vi "Backup.vi"() -> ()   [LabVIEW 2020, in "Backup.lvlib"]
uses:
  Backup.lvlib
  Seiten/System Einstellungen V2/Aktioen FGV System Konstanten.ctl
  Sprachverwaltung/FGV Aktion Tabelle zerlegen.ctl
  Seiten/FT-IR/Span/Aktion FGV Span.ctl
  Bildwechsel/Bild-Auswahl.ctl
  <vilib>/Platform/browser.llb/Open URL in Default Browser (path).vi
  Allgemein/allgemeine Sub-VIs.lvlib
  Seiten/System Einstellungen V2/System Einstellungen V2.lvlib
  Bildwechsel/Bildwechsel.lvlib
  Seiten/FT-IR/Span/Spanfaktor.lvlib
  Sprachverwaltung/Sprachverwaltung.lvlib
panel:
  out "Statusanzeige":string
  out "SysLog":bool
  out "recipes":bool caption="Rezepte"
  out "Communication":bool caption="Kommunikation"
  out "cRIO KonfigIAG":bool
  out "cRIO startup":bool
  in  "Listenfeld":i32(listbox)
  in  "Cancel":bool
  in  "Backup":bool caption="Update"
  # "Backup Manager"
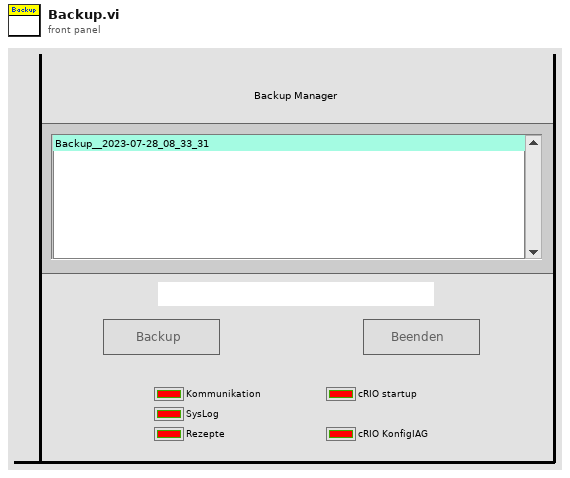
[diagram p1: front panel]
types:
  T1 = typedef "Sprachverwaltung.lvlib/FGV Aktion Tabelle zerlegen.ctl" = enum16{"laden", "vereinzeln", "speichern"}
  T2 = enum8{"Enabled", "Disabled", "Disabled and Grayed Out"}
  T3 = typedef "System Einstellungen V2.lvlib/Aktioen FGV System Konstanten.ctl" = enum16{"lesen", "laden", "speichern", "Sprache"}
  T4 = typedef "FT-IR.lvlib/Spanfaktor.lvlib/Aktion FGV Span.ctl" = enum16{"lesen", "Span", "Seite aktiv", "Offset", "FGV aktualisiert", "Aktualisierung aufheben"}
  T5 = typedef "Bildwechsel.lvlib/Bild-Auswahl.ctl" = enum16{"lesen", "Initialisieren", "Beenden", "Grafik", "Anlagenübersicht", "Anlagengrenzwerte", "Log Konfig", "Gaszuordnung AO", "Erw. Konfiguration", "FT-IR  ", "Störmeldungen", "Störmeldepuffer", "Störmeldekonfig", "PNS Grenzwerte", "Statusübersicht", "Linearisierung", "ARN", "EPA Dichtheitstest", "FID", "PMA", "CalGas", "Lambda", "Interference", "Amium PNS", "EPA T90", "Interference N2O", "Scheduler", "Systemeinstellungen", "EPA Drift", "CAN Konfig"}
  T6 = cluster{"Modell":string, "ProjektNummer":string, "Software Version":string, "Seriennummer":string}
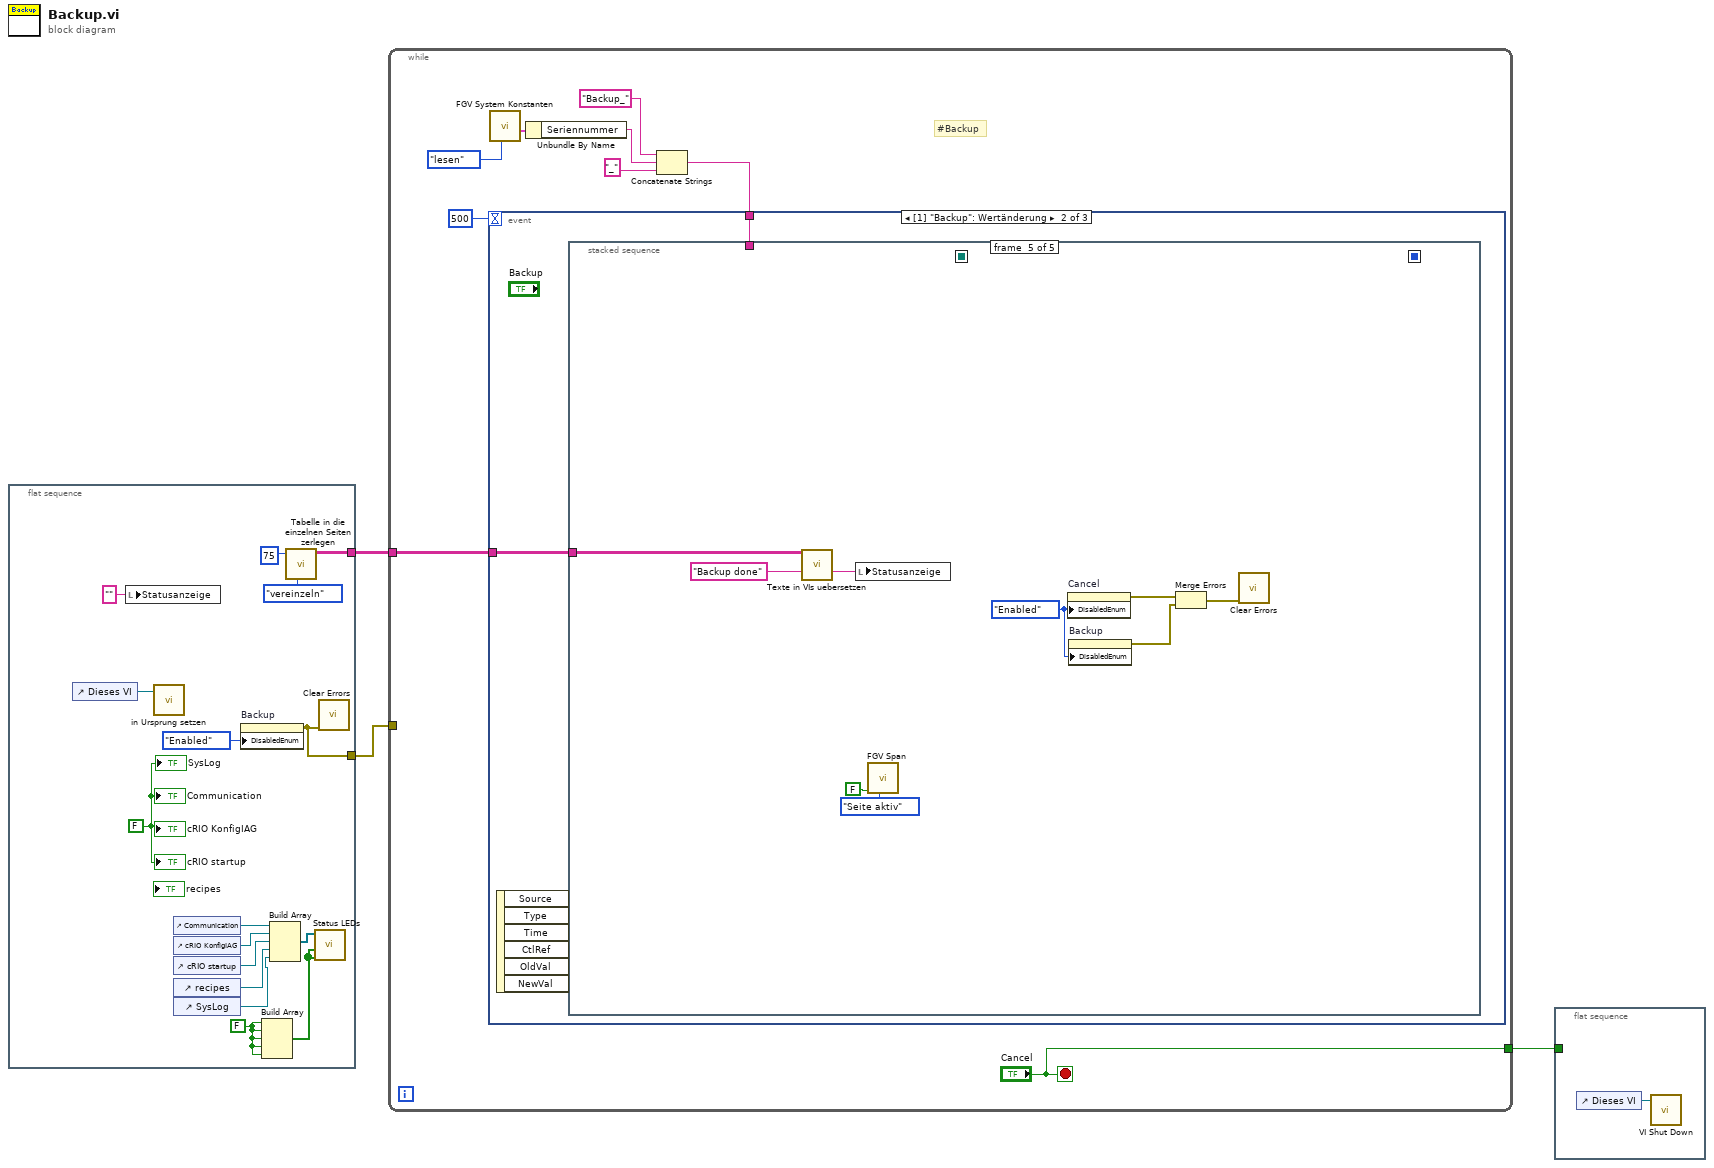
[diagram p0: block diagram]
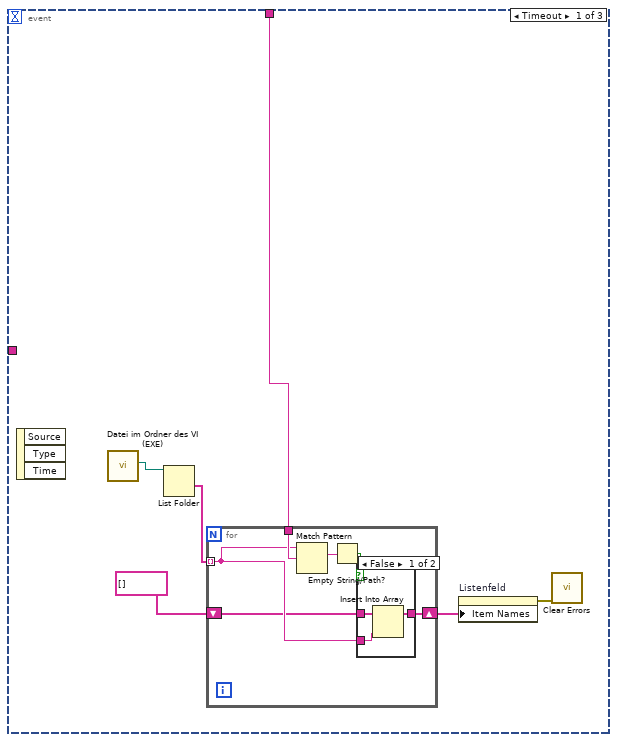
[diagram p2: hidden frame]
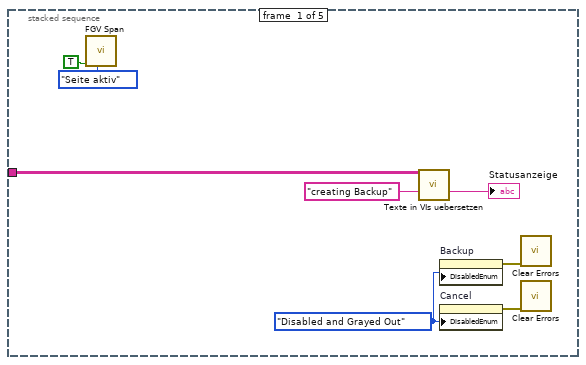
[diagram p4: hidden frame]
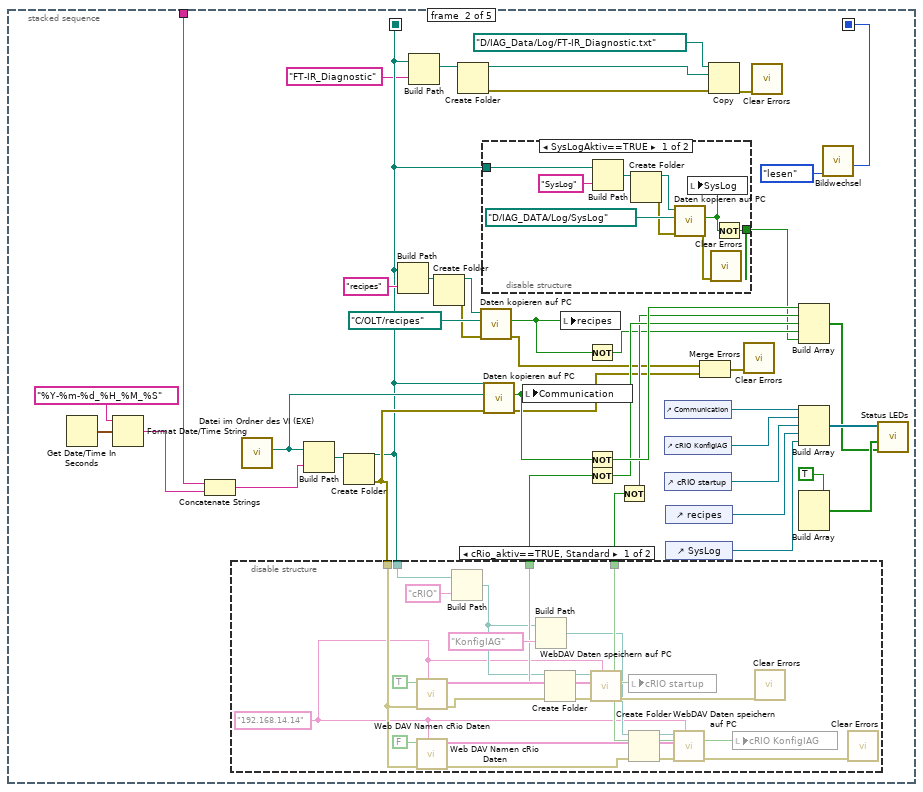
[diagram p5: hidden frame]
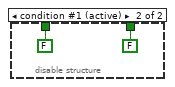
[diagram p7: hidden frame]
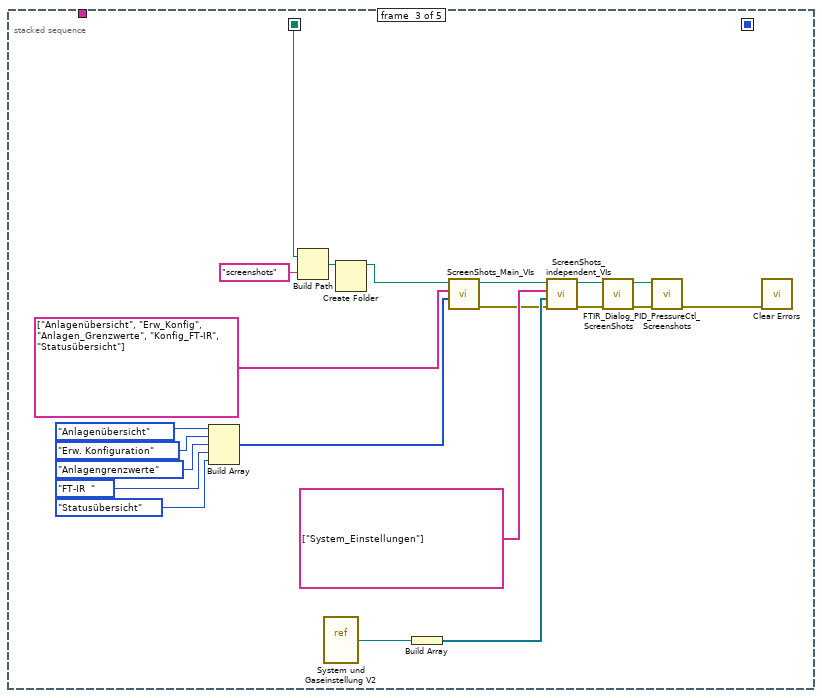
[diagram p8: hidden frame]
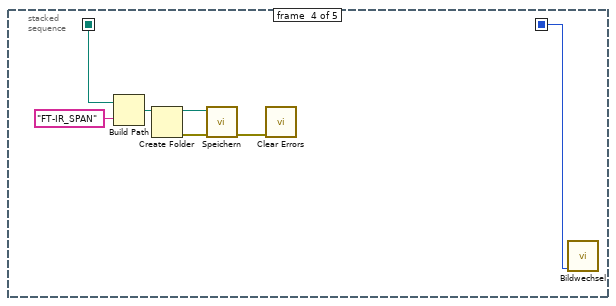
[diagram p9: hidden frame]
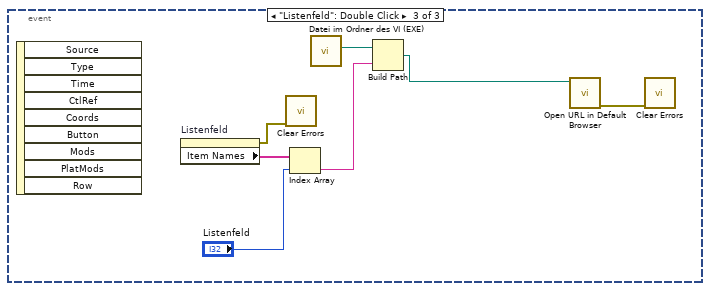
[diagram p10: hidden frame]
diagram:
  n1 = flat-sequence {
    tunnel: [w18] -> w2
    tunnel: [w5] -> w1
    frame #0 {
      w8 = FALSE
      w10 = FALSE
      n2 = control-ref of="Dieses VI"() -> (w12:refnum<vi>)
      n3 = local write "Statusanzeige"("" ("Statusanzeige")) -> ()
      n4 = call "in Ursprung setzen.vi"("VI Referenz"=w12) -> ()  [unwired: 10 in, 1 out]
      n5 = control-ref of="Communication"() -> (w17:refnum<vi>)
      n6 = control-ref of="cRIO KonfigIAG"() -> (w16:refnum<vi>)
      n7 = control-ref of="cRIO startup"() -> (w15:refnum<vi>)
      n8 = control-ref of="recipes"() -> (w11:refnum<vi>)
      n9 = control-ref of="SysLog"() -> (w9:refnum<vi>)
      n10 = property on="Backup" class="Bool."("DisabledEnum"=T2."Enabled" ("Deaktiviert")) -> (error out=w18:errorcluster)  [unwired: 2 in, 1 out]
      n11 = Build Array(w8, w8, w8, w8, w8) -> (w13:bool[])
      n12 = Build Array(w17, w16, w15, w11, w9) -> (w14:refnum<vi>[])
      n13 = call "Tabelle in die einzelnen Seiten zerlegen.vi"("Aktion"=FGV_Aktion_Tabelle_zerlegen."vereinzeln", "Index (Seite)"=75) -> ("Sprachliste"=w5:string[][])  [unwired: 7 in, 2 out]
      n14 = call "Status LEDs.vi"("Array Error"=w13, "Array Aktiv"=w13, "Array LED"=w14) -> ()  [unwired: 9 in]
      n15 = call <vilib>:"Clear Errors.vi"("error in (no error)"=w18) -> ()  [unwired: 5 in, 2 out]
      "Communication" <- w10
      "cRIO startup" <- w10
      "cRIO KonfigIAG" <- w10
      "SysLog" <- w10
    }
  }
  n16 = while {
    tunnel: ["Cancel"] -> w3
    tunnel: w2 -> [_]
    tunnel: w1 -> [w20]
    stop <- "Cancel" stop-if-true
    # "#Backup"
    n17 = call "FGV System Konstanten.vi"("Aktionen"=Aktioen_FGV_System_Konstanten."lesen") -> ("Cluster out"=w22:T6)  [unwired: 6 in, 4 out]
    n18 = Unbundle By Name(w22) -> ("Seriennummer"=w21:string)
    n19 = Concatenate Strings("Backup_" ("String"), w21, "_" ("String")) -> (w23:string)
    n20 = event shown="[1] \"Backup\": Wertänderung" {
      selector: _ -> [_ _ _]
      dyn-events: _ -> [_ _ _]
      timeout: 500 -> [_ _ _]
      tunnel: w23 -> [w29 w46 _]
      tunnel: w20 -> [_ w45 _]
      event Timeout {
        n21 = event-data() -> ()  [unwired: 1 in, 3 out]
        n22 = call "Datei im Ordner des VI (EXE).vi"() -> ("Ordner des Haupt-VIs"=w34:path)  [unwired: 9 in, 2 out]
        n23 = List Folder(path=w34) -> (folder names=w30:string[])  [unwired: 3 in, 3 out]
        n24 = for {
          tunnel: w30 -> [w37] mode=indexing
          tunnel: w29 -> [w40]
          shift-right: [w35] -> w32
          shift-left: string[] [] -> [w36]
          n25 = Match Pattern(string=w37, regular expression=w40) -> (match substring=w39:string)  [unwired: 1 in, 3 out]
          n26 = Empty String/Path?(string/path=w39) -> (empty?=w38:bool)
          n27 = case shown="False" w38 {
            tunnel: w37 -> [w42 _]
            tunnel: w36 -> [w43 w44]
            tunnel: [w41 w44] -> w35
            frame False {
              n28 = Insert Into Array(array=w43, new element=w42) -> (w41:string[])  [unwired: 1 in]
            }
            frame True {
            }
          }
        }
        n29 = property on="Listenfeld" class="Listenfeld (strikt)"("Item Names"=w32) -> (error out=w31:errorcluster)  [unwired: 2 in, 1 out]
        n30 = call <vilib>:"Clear Errors.vi"("error in (no error)"=w31) -> ()  [unwired: 5 in, 2 out]
      }
      event "Backup": Value Change {
        n31 = event-data() -> ()  [unwired: 1 in, 6 out]
        n32 = stacked-sequence {
          seq-local: [_ w62 _ _ _] -> [_ _ w148 w154 _]
          seq-local: [_ w66 _ _ _] -> [_ _ _ w157 _]
          tunnel: w46 -> [_ w79 _ _ _]
          tunnel: w45 -> [w47 _ _ _ w159]
          frame #0 {
            w53 = T2."Disabled and Grayed Out" ("Deaktiviert")
            n33 = call "FGV Span.vi"("Aktion"=Aktion_FGV_Span."Seite aktiv", "Aktiv"=TRUE) -> ()  [unwired: 6 in, 4 out]
            n34 = call "Texte in VIs uebersetzen.vi"("Sprachliste"=w47, "String zum Übersetzen"="creating Backup") -> ("String zum Übersetzen"=→"Statusanzeige":string)  [unwired: 9 in, 4 out]
            n35 = property on="Backup" class="Bool."("DisabledEnum"=w53) -> (error out=w54:errorcluster)  [unwired: 2 in, 1 out]
            n36 = property on="Cancel" class="Bool."("DisabledEnum"=w53) -> (error out=w52:errorcluster)  [unwired: 2 in, 1 out]
            n37 = call <vilib>:"Clear Errors.vi"("error in (no error)"=w54) -> ()  [unwired: 5 in, 2 out]
            n38 = call <vilib>:"Clear Errors.vi"("error in (no error)"=w52) -> ()  [unwired: 5 in, 2 out]
          }
          frame #1 {
            w64 = TRUE
            n39 = Get Date/Time In Seconds() -> (seconds since 1Jan1904=w97:timestamp)
            n40 = Format Date/Time String(time format string (%c)="%Y-%m-%d_%H_%M_%S" ("Format-String"), seconds (now)=w97) -> (date/time string=w81:string)  [unwired: 1 in]
            n41 = Concatenate Strings(w79, w81) -> (w80:string)
            n42 = call "Datei im Ordner des VI (EXE).vi"() -> ("Ordner des Haupt-VIs"=w68:path)  [unwired: 9 in, 2 out]
            n43 = Build Path(base path=w68, name or relative path=w80) -> (appended path=w95:path)
            n44 = Create Folder(path (use dialog)=w95) -> (created path=w62:path, error out=w94:errorcluster)  [unwired: 2 in, 1 out]
            n45 = disable-structure shown="cRio_aktiv==TRUE, Standard" {
              disable-tunnel: w62 -> [w121 _]
              disable-tunnel: w94 -> [w120 _]
              disable-tunnel: [w117 FALSE ("ohne Fehler")] -> w86
              disable-tunnel: [w116 FALSE ("ohne Fehler")] -> w84
              frame condition #0 {
                w107 = "192.168.14.14" ("IP Adresse")
                n46 = call "Web DAV Namen cRio Daten.vi"("IP Adresse"=w107, "error in"=w120, "startup"=TRUE) -> ("error out"=w113:errorcluster, "Dateien FTP"=w123:string[])  [unwired: 6 in, 1 out]
                n47 = call "Web DAV Namen cRio Daten.vi"("IP Adresse"=w107, "error in"=w120, "startup"=FALSE) -> ("error out"=w109:errorcluster, "Dateien FTP"=w122:string[])  [unwired: 6 in, 1 out]
                n48 = Build Path(base path=w121, name or relative path="cRIO" ("String")) -> (appended path=w115:path)
                n49 = Build Path(base path=w115, name or relative path="KonfigIAG" ("String")) -> (appended path=w111:path)
                n50 = Create Folder(path (use dialog)=w115, error in=w113) -> (created path=w114:path, error out=w112:errorcluster)  [unwired: 1 in, 1 out]
                n51 = call "WebDAV Daten speichern auf PC.vi"("IP Adresse"=w107, "error in"=w112, "Dateinamen"=w123, "Pfad PC"=w114) -> ("error out"=w119:errorcluster, "ohne Fehler"=w117:bool)  [unwired: 6 in]
                n52 = local write "cRIO startup"(w117) -> ()
                n53 = Create Folder(path (use dialog)=w111, error in=w109) -> (created path=w110:path, error out=w108:errorcluster)  [unwired: 1 in, 1 out]
                n54 = call "WebDAV Daten speichern auf PC.vi"("IP Adresse"=w107, "error in"=w108, "Dateinamen"=w122, "Pfad PC"=w110) -> ("error out"=w118:errorcluster, "ohne Fehler"=w116:bool)  [unwired: 6 in]
                n55 = local write "cRIO KonfigIAG"(w116) -> ()
                n56 = call <vilib>:"Clear Errors.vi"("error in (no error)"=w119) -> ()  [unwired: 5 in, 2 out]
                n57 = call <vilib>:"Clear Errors.vi"("error in (no error)"=w118) -> ()  [unwired: 5 in, 2 out]
              }
              frame condition #1 (active) {
              }
            }
            n58 = Build Path(base path=w62, name or relative path="recipes" ("Name oder relativer Pfad")) -> (appended path=w71:path)
            n59 = Build Path(base path=w62, name or relative path="FT-IR_Diagnostic") -> (appended path=w60:path)
            n60 = Create Folder(path (use dialog)=w71) -> (created path=w70:path, error out=w59:errorcluster)  [unwired: 2 in, 1 out]
            n61 = Create Folder(path (use dialog)=w60) -> (created path=w55:path, error out=w57:errorcluster)  [unwired: 2 in, 1 out]
            n62 = call "Daten kopieren auf PC.vi"("error in"=w59, "Pfad Communication"=path "C:/OLT/recipes", "Pfad PC"=w70) -> ("error out"=w77:errorcluster, "ohne Fehler"=w74:bool)  [unwired: 7 in]
            n63 = disable-structure shown="SysLogAktiv==TRUE" {
              disable-tunnel: w62 -> [w102 _]
              disable-tunnel: [w100 _] -> w63
              frame condition #0 (active) {
                n64 = Build Path(base path=w102, name or relative path="SysLog" ("Name oder relativer Pfad")) -> (appended path=w105:path)
                n65 = Create Folder(path (use dialog)=w105) -> (created path=w104:path, error out=w98:errorcluster)  [unwired: 2 in, 1 out]
                n66 = call "Daten kopieren auf PC.vi"("error in"=w98, "Pfad Communication"=path "D:/IAG_DATA/Log/SysLog", "Pfad PC"=w104) -> ("error out"=w99:errorcluster, "ohne Fehler"=w101:bool)  [unwired: 7 in]
                n67 = local write "SysLog"(w101) -> ()
                n68 = call <vilib>:"Clear Errors.vi"("error in (no error)"=w99) -> ()  [unwired: 5 in, 2 out]
                n69 = Not(x=w101) -> (.not. x?=w100:bool)
              }
              frame condition #1 {
              }
            }
            n70 = call "Daten kopieren auf PC.vi"("error in"=w94, "Pfad Communication"=w68, "Pfad PC"=w62) -> ("error out"=w76:errorcluster, "ohne Fehler"=w88:bool)  [unwired: 7 in]
            n71 = local write "Communication"(w88) -> ()
            n72 = local write "recipes"(w74) -> ()
            n73 = Not(x=w74) -> (.not. x?=w73:bool)
            n74 = Not(x=w88) -> (.not. x?=w87:bool)
            n75 = Not(x=w86) -> (.not. x?=w85:bool)
            n76 = Not(x=w84) -> (.not. x?=w83:bool)
            n77 = control-ref of="Communication"() -> (w93:refnum<vi>)
            n78 = control-ref of="cRIO KonfigIAG"() -> (w92:refnum<vi>)
            n79 = control-ref of="cRIO startup"() -> (w91:refnum<vi>)
            n80 = control-ref of="recipes"() -> (w72:refnum<vi>)
            n81 = control-ref of="SysLog"() -> (w65:refnum<vi>)
            n82 = Merge Errors(w77, w76) -> (w78:errorcluster)
            n83 = Copy(8:w57, 10:w55, 11:path "D:/IAG_Data/Log/FT-IR_Diagnostic.txt" ("Pfad Communication")) -> (0:w58:errorcluster)  [unwired: 2 in, 2 out]
            n84 = call <vilib>:"Clear Errors.vi"("error in (no error)"=w78) -> ()  [unwired: 5 in, 2 out]
            n85 = call <vilib>:"Clear Errors.vi"("error in (no error)"=w58) -> ()  [unwired: 5 in, 2 out]
            n86 = Build Array(w87, w83, w85, w73, w63) -> (w82:bool[])
            n87 = Build Array(w93, w92, w91, w72, w65) -> (w90:refnum<vi>[])
            n88 = Build Array(w64, w64, w64, w64, w64) -> (w89:bool[])
            n89 = call "Bildwechsel.vi"("nächstes Bild"=Bild-Auswahl."lesen") -> ("aktuelle Bildnummer"=w66:T5)  [unwired: 9 in, 1 out]
            n90 = call "Status LEDs.vi"("Array Error"=w82, "Array Aktiv"=w89, "Array LED"=w90) -> ()  [unwired: 9 in]
          }
          frame #2 {
            n91 = Build Array(Bild-Auswahl."Anlagenübersicht" ("Bild-Auswahl"), Bild-Auswahl."Erw. Konfiguration" ("Bild-Auswahl"), Bild-Auswahl."Anlagengrenzwerte" ("Bild-Auswahl"), Bild-Auswahl."FT-IR  " ("Bild-Auswahl"), Bild-Auswahl."Statusübersicht" ("Bild-Auswahl")) -> (w134:T5[])
            n92 = Build Path(base path=w148, name or relative path="screenshots" ("Name oder relativer Pfad")) -> (appended path=w150:path)
            n93 = vi-ref "System und Gaseinstellung V2.vi"() -> (w146:refnum<vi>)
            n94 = Create Folder(path (use dialog)=w150) -> (created path=w137:path)  [unwired: 2 in, 2 out]
            n95 = Build Array(w146) -> (w145:refnum<vi>[])
            n96 = call "ScreenShots_Main_VIs.vi"("Bild Auswahl"=w134, "filename"=string[] ["Anlagenübersicht", "Erw_Konfig", "Anlagen_Grenzwerte", "Konfig_FT-IR", "Statusübersicht"], "Screenshots Pfad"=w137) -> ("error out"=w135:errorcluster, "Screenshots Pfad out"=w136:path)  [unwired: 7 in]
            n97 = call "ScreenShots_independent_VIs.vi"("error in"=w135, "referenz"=w145, "filename"=string[] ["System_Einstellungen"], "Screenshots Pfad"=w136) -> ("error out"=w144:errorcluster, "Screenshots Pfad  out"=w143:path)  [unwired: 6 in]
            n98 = call "FTIR_Dialog_ScreenShots.vi"("error in"=w144, "Screenshots Pfad"=w143) -> ("error out"=w131:errorcluster, "Screenshots Pfad  out"=w132:path)  [unwired: 8 in]
            n99 = call "PID_PressureCtl_Screenshots.vi"("error in"=w131, "Screenshots Pfad"=w132) -> ("error out 2"=w130:errorcluster)  [unwired: 8 in, 1 out]
            n100 = call <vilib>:"Clear Errors.vi"("error in (no error)"=w130) -> ()  [unwired: 5 in, 2 out]
          }
          frame #3 {
            n101 = Build Path(base path=w154, name or relative path="FT-IR_SPAN" ("Name oder relativer Pfad")) -> (appended path=w155:path)
            n102 = Create Folder(path (use dialog)=w155) -> (created path=w151:path, error out=w153:errorcluster)  [unwired: 2 in, 1 out]
            n103 = call "Speichern.vi"("Fehler (Eingang)"=w153, "pfad"=w151) -> ("Fehler (Ausgang)"=w152:errorcluster)  [unwired: 9 in]
            n104 = call <vilib>:"Clear Errors.vi"("error in (no error)"=w152) -> ()  [unwired: 5 in, 2 out]
            n105 = call "Bildwechsel.vi"("nächstes Bild"=w157) -> ()  [unwired: 9 in, 2 out]
          }
          frame #4 {
            w161 = T2."Enabled" ("Deaktiviert")
            n106 = call "Texte in VIs uebersetzen.vi"("Sprachliste"=w159, "String zum Übersetzen"="Backup done") -> ("String zum Übersetzen"=w158:string)  [unwired: 9 in, 4 out]
            n107 = local write "Statusanzeige"(w158) -> ()
            n108 = call "FGV Span.vi"("Aktion"=Aktion_FGV_Span."Seite aktiv", "Aktiv"=FALSE) -> ()  [unwired: 6 in, 4 out]
            n109 = property on="Cancel" class="Bool."("DisabledEnum"=w161) -> (error out=w164:errorcluster)  [unwired: 2 in, 1 out]
            n110 = property on="Backup" class="Bool."("DisabledEnum"=w161) -> (error out=w163:errorcluster)  [unwired: 2 in, 1 out]
            n111 = Merge Errors(w164, w163) -> (w162:errorcluster)
            n112 = call <vilib>:"Clear Errors.vi"("error in (no error)"=w162) -> ()  [unwired: 5 in, 2 out]
          }
        }
      }
      event "Listenfeld": Double Click {
        n113 = event-data() -> ()  [unwired: 1 in, 9 out]
        n114 = property on="Listenfeld" class="Listenfeld (strikt)"() -> (error out=w171:errorcluster, "Item Names"=w173:string[])  [unwired: 2 in, 1 out]
        n115 = call <vilib>:"Clear Errors.vi"("error in (no error)"=w171) -> ()  [unwired: 5 in, 2 out]
        n116 = Index Array(array=w173, index="Listenfeld") -> (element=w168:string)
        n117 = call "Datei im Ordner des VI (EXE).vi"() -> ("Ordner des Haupt-VIs"=w169:path)  [unwired: 9 in, 2 out]
        n118 = Build Path(base path=w169, name or relative path=w168) -> (appended path=w167:path)
        n119 = call-poly <vilib>:"Open URL in Default Browser.vi"("path"=w167) -> ("error out"=w170:errorcluster)  [unwired: 5 in, 1 out]
        n120 = call <vilib>:"Clear Errors.vi"("error in (no error)"=w170) -> ()  [unwired: 5 in, 2 out]
      }
    }
  }
  n121 = flat-sequence {
    tunnel: w3 -> [_]
    frame #0 {
      n122 = control-ref of="Dieses VI"() -> (w174:refnum<vi>)
      n123 = call "VI Shut Down.vi"("VI Referenz"=w174) -> ()  [unwired: 11 in]
    }
  }
